vi "Read State.vi"(9 "String (T)":bool=TRUE, 11 "Interlock in":refnum<class "Interlock.lvclass">) -> (1 "State string":string, 2 "State":T1, 3 "Interlock out":refnum<class "Interlock.lvclass">)   [LabVIEW 2015, in "Interlocks.lvlib" / "Interlock.lvclass"]
uses:
  Interlock.lvclass
  State Enum.ctl
  Interlock.lvclass/Interlock.ctl
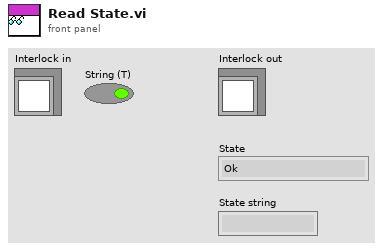
[diagram p1: front panel]
types:
  T1 = typedef "Interlocks.lvlib/Interlock.lvclass/State Enum.ctl" = enum16{"Ok", "Interlock", "Out of Range", "Is ON", "Is OFF", "Error", "Denied", "Not Allowed", "Sample Allow", "Sample Deny"}
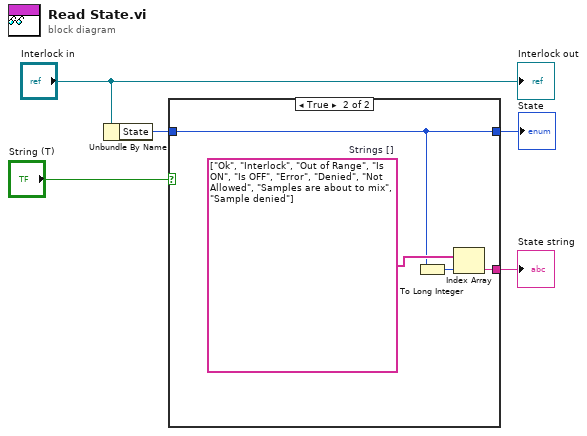
[diagram p0: block diagram]
diagram:
  n1 = Unbundle By Name("Interlock in") -> ("State"=w2:T1)
  n2 = case shown="True" "String (T)" {
    tunnel: [_ w9] -> w4
    tunnel: w2 -> [w6 w7]
    tunnel: [w6 w7] -> w1
    frame False {
    }
    frame True {
      w8 = string[] ["Ok", "Interlock", "Out of Range", "Is ON", "Is OFF", "Error", "Denied", "Not Allowed", "Samples are about to mix", "Sample denied"]  # Strings []
      n3 = To Long Integer(number=w7) -> (32bit integer=w10:i32)
      n4 = Index Array(array=w8, index=w10) -> (element=w9:string)
    }
  }
  "State" <- w1
  "State string" <- w4
  "Interlock out" <- "Interlock in"
